vi "载波.vi"(1 "相位输入":dbl, 2 "载频":dbl, 3 "采样率":dbl, 4 "采样点数":i32=128 caption="采样点数N") -> (0 "载波信号波形":dbl[](array[numeric]) caption="正弦信号")   [LabVIEW 2013]
uses:
  <vilib>/Analysis/NI_AALBase.lvlib
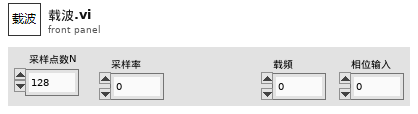
[diagram p1: front panel]
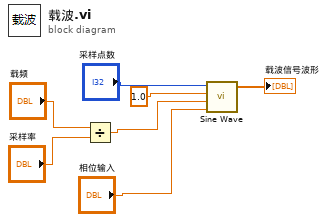
[diagram p0: block diagram]
diagram:
  n1 = Divide(x="载频", y="采样率") -> (x/y=w3:dbl)
  n2 = call <vilib>:"Sine Wave.vi"("samples"="采样点数", "amplitude"=1.0, "frequency"=w3, "phase in"="相位输入") -> ("sine wave"=→"载波信号波形":dbl[])  [unwired: 1 in, 2 out]
